vi "ChannelType_1D-Array-U16.vi"(9 "error in":errorcluster, 11 "Array in":u16[](array[numeric])) -> (1 "error out":errorcluster, 2 "ChannelType":u16, 3 "Array out":u16[](array[numeric]))   [LabVIEW 2020, in "OpenLvVision_OpenCv.lvlib"]
uses:
  OpenLvVision_OpenCv.lvlib
  <vilib>/Utility/error.llb/Error Cluster From Error Code.vi
  <vilib>/ErrorRing/Error Ring.xnode
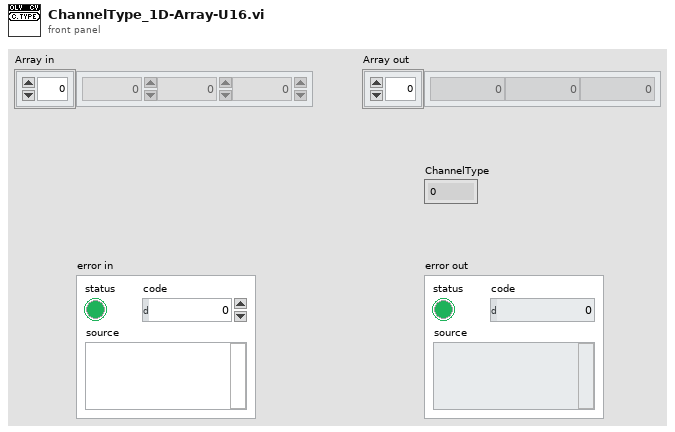
[diagram p1: front panel]
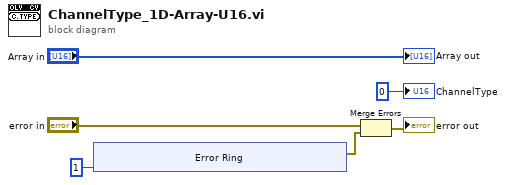
[diagram p0: block diagram]
diagram:
  n1 = xnode "Error Ring"("parameter 0"=1) -> ("error out"=w2:errorcluster)
  n2 = Merge Errors("error in", w2) -> (→"error out":errorcluster)
  "Array out" <- "Array in"
  "ChannelType" <- u16 0
